vi "Read Color.vi"(11 "Piece in":refnum<class "Piece.lvclass">) -> (2 "Color":T1)   [LabVIEW 2015, in "Chesslib.lvlib" / "Piece.lvclass"]
uses:
  Piece.lvclass
  typedef/Color.ctl
  Piece.lvclass/Piece.ctl
  Chesslib.lvlib
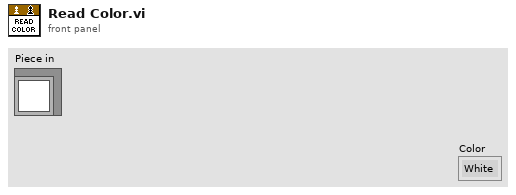
[diagram p1: front panel]
types:
  T1 = typedef "Chesslib.lvlib/Color.ctl" = enum16{"White", "Black"}
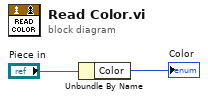
[diagram p0: block diagram]
diagram:
  n1 = Unbundle By Name("Piece in") -> ("Color"=→"Color":T1)
